vi "CalculateWallPose.vi"(8 "Lidar Angles":dbl[](array[numeric])=[-99.9609375, -99.609375, -99.2578125, -98.90625, -98.5546875, -98.203125, -97.8515625, -97.5, -97.1484375, -96.796875, -96.4453125, -96.09375, -95.7421875, -95.390625, -95.0390625, -94.6875, -94.3359375, -93.984375, -93.6328125, -93.28125, -92.9296875, -92.578125, -92.2265625, -91.875, -91.5234375, -91.171875, -90.8203125, -90.46875, -90.1171875, -89.765625, -89.4140625, -89.0625, -88.7109375, -88.359375, -88.0078125, -87.65625, -87.3046875, -86.953125, -86.6015625, -86.25, -85.8984375, -85.546875, -85.1953125, -84.84375, -84.4921875, -84.140625, -83.7890625, -83.4375, -83.0859375, -82.734375, -82.3828125, -82.03125, -81.6796875, -81.328125, -80.9765625, -80.625, -80.2734375, -79.921875, -79.5703125, -79.21875, -78.8671875, -78.515625, -78.1640625, -77.8125, -77.4609375, -77.109375, -76.7578125, -76.40625, -76.0546875, -75.703125, -75.3515625, -75.0, -74.6484375, -74.296875, -73.9453125, -73.59375, -73.2421875, -72.890625, -72.5390625, -72.1875, -71.8359375, -71.484375, -71.1328125, -70.78125, -70.4296875, -70.078125, -69.7265625, -69.375, -69.0234375, -68.671875, -68.3203125, -67.96875, -67.6171875, -67.265625, -66.9140625, -66.5625, -66.2109375, -65.859375, -65.5078125, -65.15625, -64.8046875, -64.453125, -64.1015625, -63.75, -63.3984375, -63.046875, -62.6953125, -62.34375, -61.9921875, -61.640625, -61.2890625, -60.9375, -60.5859375, -60.234375, -59.8828125, -59.53125, -59.1796875, -58.828125, -58.4765625, -58.125, -57.7734375, -57.421875, -57.0703125, -56.71875, -56.3671875, -56.015625, -55.6640625, -55.3125, -54.9609375, -54.609375, -54.2578125, -53.90625, -53.5546875, -53.203125, -52.8515625, -52.5, -52.1484375, -51.796875, -51.4453125, -51.09375, -50.7421875, -50.390625, -50.0390625, -49.6875, -49.3359375, -48.984375, -48.6328125, -48.28125, -47.9296875, -47.578125, -47.2265625, -46.875, -46.5234375, -46.171875, -45.8203125, -45.46875, -45.1171875], 9 "Lidar Magnitude":dbl[](array[numeric])=[372.0, 372.0, 372.0, 372.0, 372.0, 373.0, 372.0, 371.0, 373.0, 371.0, 371.0, 371.0, 378.0, 375.0, 377.0, 380.0, 380.0, 377.0, 378.0, 378.0, 376.0, 370.0, 373.0, 372.0, 369.0, 369.0, 371.0, 371.0, 371.0, 372.0, 372.0, 378.0, 372.0, 371.0, 371.0, 370.0, 370.0, 370.0, 369.0, 369.0, 369.0, 369.0, 369.0, 369.0, 376.0, 376.0, 376.0, 366.0, 375.0, 366.0, 371.0, 371.0, 375.0, 372.0, 375.0, 378.0, 378.0, 378.0, 378.0, 378.0, 376.0, 375.0, 375.0, 375.0, 378.0, 378.0, 378.0, 378.0, 378.0, 380.0, 380.0, 378.0, 377.0, 377.0, 377.0, 377.0, 377.0, 378.0, 382.0, 382.0, 383.0, 383.0, 383.0, 383.0, 387.0, 387.0, 387.0, 387.0, 387.0, 388.0, 389.0, 391.0, 393.0, 393.0, 393.0, 396.0, 398.0, 398.0, 399.0, 399.0, 399.0, 399.0, 400.0, 399.0, 400.0, 401.0, 401.0, 403.0, 405.0, 405.0, 406.0, 406.0, 412.0, 411.0, 412.0, 413.0, 421.0, 414.0, 419.0, 419.0, 419.0, 419.0, 424.0, 424.0, 426.0, 433.0, 429.0, 429.0, 433.0, 429.0, 429.0, 436.0, 437.0, 442.0, 443.0, 443.0, 449.0, 451.0, 451.0, 451.0, 457.0, 459.0, 457.0, 459.0, 460.0, 465.0, 467.0, 472.0, 472.0, 478.0, 478.0, 478.0, 479.0, 485.0, 485.0, 485.0, 496.0], 11 "Wall Left?":bool=TRUE) -> (0 "Angle to Wall":dbl, 1 "Error":dbl=368.4, 3 "OH SHIT NO LIDAR DATA!!!":bool)   [LabVIEW 2016]
uses:
  <vilib>/Analysis/baseanly.llb/Mean (DBL).vi
  <vilib>/Analysis/NI_AALBase.lvlib
panel:
  in  "Desired Angle 2":dbl=-57.0
  in  "Desired Angle":dbl=-80.0
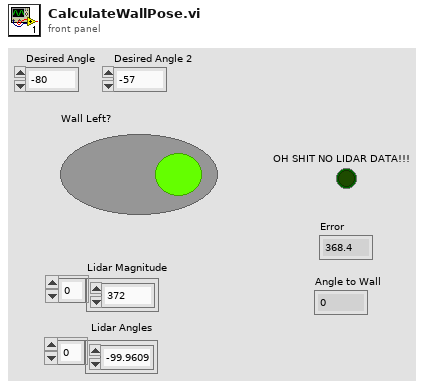
[diagram p1: front panel]
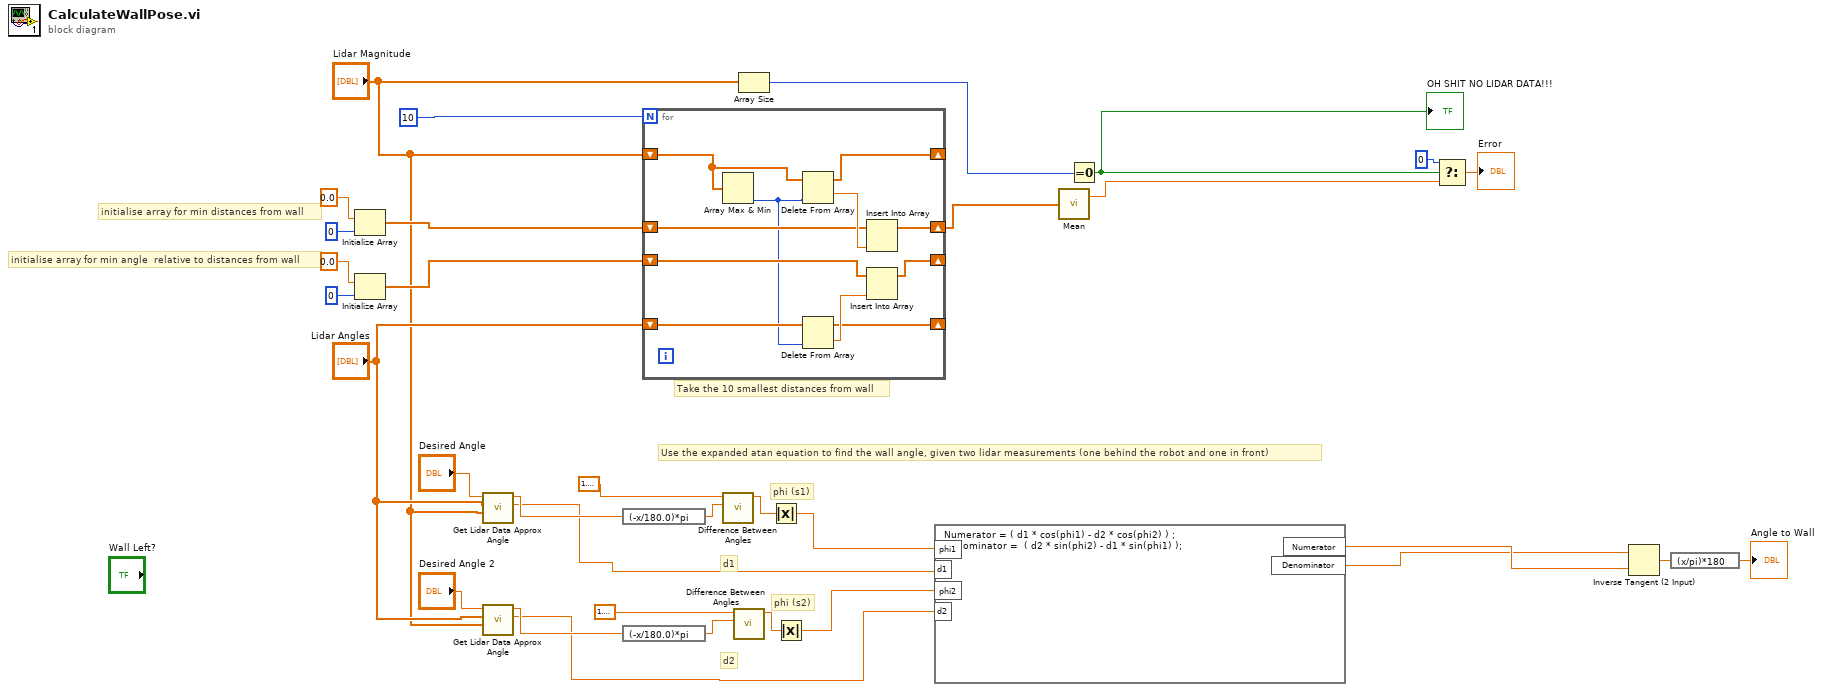
[diagram p0: block diagram]
diagram:
  # "d2"
  # "phi (s1)"
  # "phi (s2)"
  # "d1"
  # "Use the expanded atan equation to find the wall angle, given two lidar measurements (one behind the robot and one in front)"
  # "Take the 10 smallest distances from wall"
  # "initialise array for min angle  relative to distances from wall"
  # "initialise array for min distances from wall"
  n1 = Initialize Array(0.0 ("element"), 0 ("dimension size")) -> (w26:dbl[])
  n2 = Initialize Array(0.0 ("element"), 0 ("dimension size")) -> (w21:dbl[])
  n3 = call "Get Lidar Data Approx Angle.vi"("Lidar magnitude data"="Lidar Magnitude", "Lidar angle data"="Lidar Angles", "Desired Angle"="Desired Angle") -> ("Magnitude"=w3:dbl, "Angle"=w4:dbl)  [unwired: 7 in]
  n4 = call "Get Lidar Data Approx Angle.vi"("Lidar magnitude data"="Lidar Magnitude", "Lidar angle data"="Lidar Angles", "Desired Angle"="Desired Angle 2") -> ("Magnitude"=w5:dbl, "Angle"=w6:dbl)  [unwired: 7 in]
  n5 = expression code="(-x/180.0)*pi" ("degrees to radians")(w4) -> (w18:dbl)
  n6 = expression code="(-x/180.0)*pi" ("degrees to radians")(w6) -> (w17:dbl)
  n7 = for {
    N: 10 -> [_]
    shift-right: [w44] -> _
    shift-left: "Lidar Magnitude" -> [w40]
    shift-right: [w42] -> w27
    shift-left: w26 -> [w41]
    shift-right: [w39] -> _
    shift-left: w21 -> [w38]
    shift-right: [w34] -> _
    shift-left: "Lidar Angles" -> [w37]
    n8 = Array Max & Min(array=w40) -> (min index (indices)=w36:i32)  [unwired: 3 out]
    n9 = Delete From Array(array=w40, index=w36) -> (deleted portion=w43:dbl, array with subset deleted=w44:dbl[])  [unwired: 1 in]
    n10 = Delete From Array(array=w37, index=w36) -> (deleted portion=w35:dbl, array with subset deleted=w34:dbl[])  [unwired: 1 in]
    n11 = Insert Into Array(array=w41, new element=w43) -> (w42:dbl[])  [unwired: 1 in]
    n12 = Insert Into Array(array=w38, new element=w35) -> (w39:dbl[])  [unwired: 1 in]
  }
  n13 = call "Difference Between Angles.vi"("Angle 2"=w18, "Angle 1"=1.5707963267948966) -> ("Difference"=w16:dbl)  [unwired: 9 in]
  n14 = call "Difference Between Angles.vi"("Angle 2"=w17, "Angle 1"=1.5707963267948966) -> ("Difference"=w15:dbl)  [unwired: 9 in]
  n15 = Array Size(array="Lidar Magnitude") -> (size(s)=w29:i32)
  n16 = Absolute Value(x=w16) -> (abs(x)=w14:dbl)
  n17 = Absolute Value(x=w15) -> (abs(x)=w13:dbl)
  n18 = formula code="Numerator = ( d1 * cos(phi1) - d2 * cos(phi2) ) ;\nDenominator =  ( d2 * sin(phi2) - d1 * sin(phi1) );"("d1"=w3, "d2"=w5, "phi1"=w14, "phi2"=w13) -> ("Numerator"=w12:dbl, "Denominator"=w11:dbl)
  n19 = call-poly <vilib>:"Mean.vi"("X"=w27) -> ("mean"=w30:dbl)  [unwired: 1 out]
  n20 = Equal To 0?(x=w29) -> (x = 0?=w33:bool)
  "OH SHIT NO LIDAR DATA!!!" <- w33
  n21 = Select(t=0, s=w33, f=w30) -> (s? t:f=→"Error":dbl)
  n22 = Inverse Tangent (2 Input)(1:w12, 2:w11) -> (0:w10:dbl)
  n23 = expression code="(x/pi)*180" ("degrees to radians")(w10) -> (→"Angle to Wall":dbl)
